vi "Wait.vi"(8 "error in (no error)":errorcluster, 10 "Wait":bool, 11 "Waiting Dialog View in":refnum<class "Waiting Dialog View.lvclass">) -> (0 "error out":errorcluster, 3 "Waiting Dialog View out":refnum<class "Waiting Dialog View.lvclass">)   [LabVIEW 2015, in "Waiting Dialog View.lvlib" / "Waiting Dialog View.lvclass"]
uses:
  Waiting Dialog View.lvclass
  UI Controller/UI Controller Messages/Hide Subpanel Msg/Hide Subpanel Msg.lvclass
  <vilib>/Utility/miscctls.llb/LVPositionTypeDef.ctl
  UI Controller/UI Controller Messages/Hide Subpanel Msg/Hide Subpanel Msg.lvclass/Hide Subpanel Msg.ctl
  <vilib>/ActorFramework/Actor/Actor.lvclass/Actor.ctl
  <vilib>/ActorFramework/Self-Addressed Msg/Self-Addressed Msg.lvclass/Self-Addressed Msg.ctl
  <vilib>/ActorFrameworkMVC/View Controller/View Controller Messages/Insert Subpanel Msg/Insert Subpanel Msg.lvclass/Insert Subpanel Msg.ctl
  <vilib>/ActorFramework/Message Enqueuer/Message Enqueuer.lvclass/Message Enqueuer.ctl
  <vilib>/ActorFrameworkMVC/View Controller/View Controller Messages/Move Subpanel Msg/Move Subpanel Msg.lvclass/Move Subpanel Msg.ctl
  <vilib>/ActorFramework/Message Enqueuer/Enqueue.vi
  <vilib>/ActorFramework/Message Priority Queue/Priority Enqueue.vi
  <vilib>/ActorFramework/Self-Addressed Msg/Self-Addressed Msg.lvclass
  <vilib>/ActorFrameworkMVC/View Controller/View Controller Messages/Insert Subpanel Msg/Insert Subpanel Msg.lvclass
  <vilib>/ActorFrameworkMVC/View Controller/View Controller Messages/Move Subpanel Msg/Move Subpanel Msg.lvclass
  <vilib>/ActorFramework/Actor/Actor.lvclass
panel:
  # "NOTICE -- YOU MUST LEAVE THIS NOTICE IN PLACE.\n\nCopyright (c) 2015, LIANG LIU Shawn.Liu.cn@gmail.com\nAll rights reserved.\n\nRedistribution and use in source and binary forms, with or without modification, are permitted provided that the following conditions are met:\n-Redistributions of source code must retain the above copyright notice, this list of conditions and the following disclaimer.\n-Redistributions in binary form must reproduce the above copyright notice, this list of conditions and the following disclaimer in the documentation and/or other materials provided with the distribution.\n-Neither the name of the eLp nor the names of its contributors may be used to endorse or promote products derived from this software without specific prior written permission.\n\nTHIS SOFTWARE IS PROVIDED BY THE COPYRIGHT HOLDERS AND CONTRIBUTORS \"AS IS\" AND ANY EXPRESS OR IMPLIED WARRANTIES, INCLUDING, BUT NOT LIMITED TO, THE IMPLIED WARRANTIES OF MERCHANTABILITY AND FITNESS FOR A PARTICULAR PURPOSE ARE DISCLAIMED. IN NO EVENT SHALL THE COPYRIGHT HOLDER OR CONTRIBUTORS BE LIABLE FOR ANY DIRECT, INDIRECT, INCIDENTAL, SPECIAL, EXEMPLARY, OR CONSEQUENTIAL DAMAGES (INCLUDING, BUT NOT LIMITED TO, PROCUREMENT OF SUBSTITUTE GOODS OR SERVICES; LOSS OF USE, DATA, OR PROFITS; OR BUSINESS INTERRUPTION) HOWEVER CAUSED AND ON ANY THEORY OF LIABILITY, WHETHER IN CONTRACT, STRICT LIABILITY, OR TORT (INCLUDING NEGLIGENCE OR OTHERWISE) ARISING IN ANY WAY OUT OF THE USE OF THIS SOFTWARE, EVEN IF ADVISED OF THE POSSIBILITY OF SUCH DAMAGE."
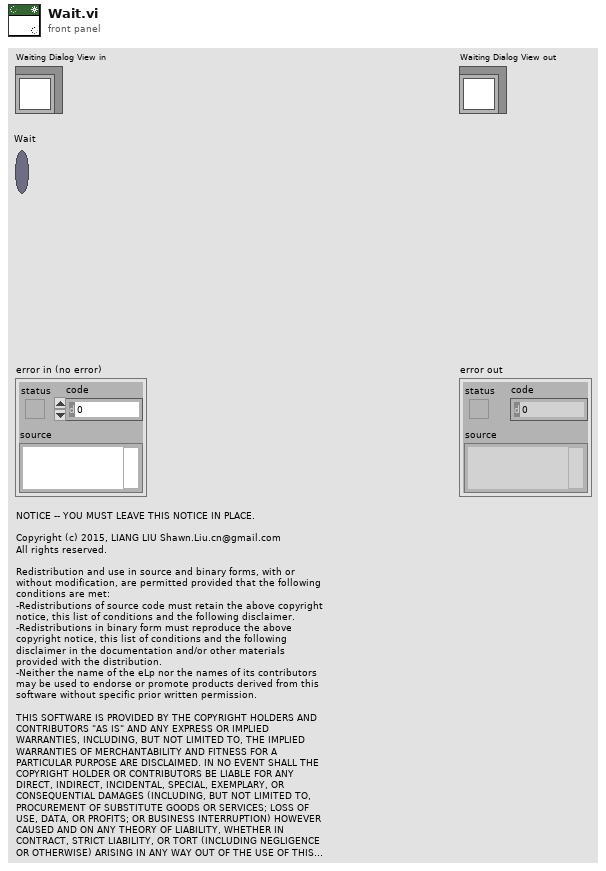
[diagram p1: front panel]
types:
  T1 = typedef "LVPositionTypeDef.ctl" = cluster{"Left":i32, "Top":i32}
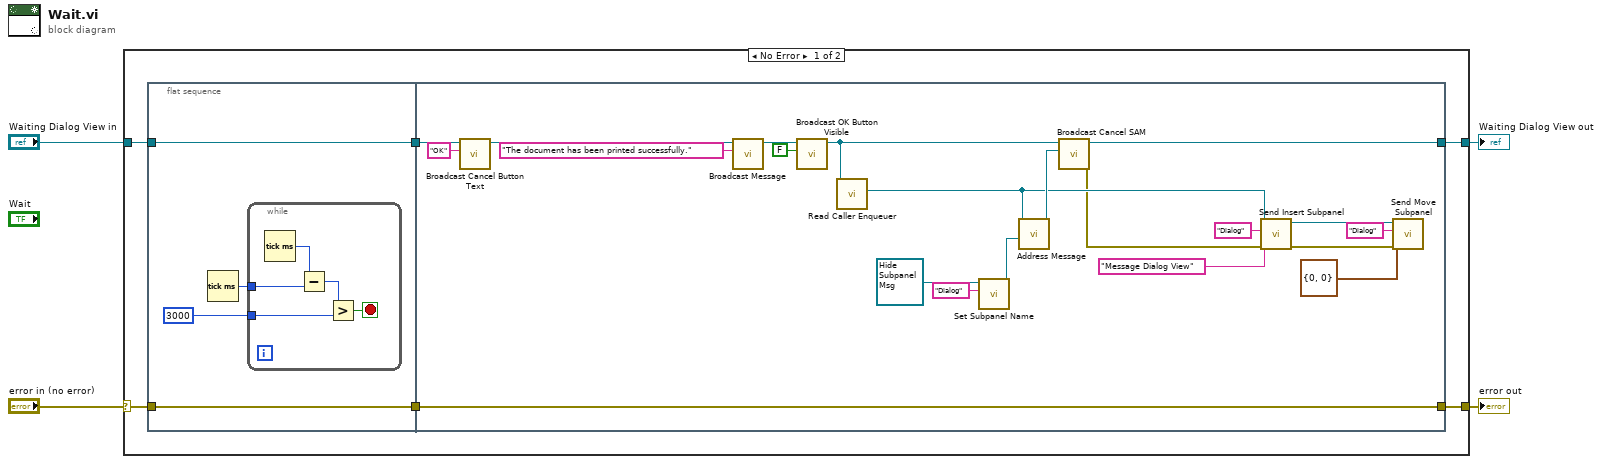
[diagram p0: block diagram]
diagram:
  n1 = case shown="No Error" "error in (no error)" {
    selector: "error in (no error)" -> [w6 w42]
    tunnel: "Waiting Dialog View in" -> [w8 w41]
    tunnel: [w7 w41] -> w3
    tunnel: [w5 w42] -> w1
    frame No Error {
      n2 = flat-sequence {
        tunnel: [w12] -> w10
        tunnel: w8 -> [w12]
        tunnel: [w11] -> w9
        tunnel: w6 -> [w11]
        tunnel: w10 -> [w40]
        tunnel: [w22] -> w7
        tunnel: w9 -> [w39]
        tunnel: [w39] -> w5
        frame #0 {
          n3 = Tick Count (ms)() -> (millisecond timer value=w14:u32)
          n4 = while {
            tunnel: w14 -> [w19]
            tunnel: u32 3000 ("y") -> [w17]
            stop <- w16 stop-if-true
            n5 = Tick Count (ms)() -> (millisecond timer value=w15:u32)
            n6 = Subtract(x=w15, y=w19) -> (x-y=w18:u32)
            n7 = Greater?(x=w18, y=w17) -> (0:w16:bool)
          }
        }
        frame #1 {
          n8 = call "Broadcast Cancel Button Text.vi"("Cancel Button Text"="OK", "Waiting Dialog View in"=w40) -> ("Waiting Dialog View out"=w38:refnum<class "Waiting Dialog View.lvclass">)  [unwired: 8 in, 1 out]
          n9 = call "Broadcast Message.vi"("Message"="The document has been printed successfully.", "Waiting Dialog View in"=w38) -> ("Waiting Dialog View out"=w36:refnum<class "Waiting Dialog View.lvclass">)  [unwired: 8 in, 1 out]
          n10 = call "Broadcast OK Button Visible.vi"("OK Button Visible"=FALSE, "Waiting Dialog View in"=w36) -> ("Waiting Dialog View out"=w23:refnum<class "Waiting Dialog View.lvclass">)  [unwired: 8 in, 1 out]
          n11 = call <vilib>:"Read Caller Enqueuer.vi"("Actor"=w23) -> ("Caller Enqueuer"=w25:refnum<class "Message Enqueuer.lvclass">)  [unwired: 10 in]
          n12 = call "Set Subpanel Name.vi"("Subpanel Name"="Dialog", "Hide Subpanel Msg in"=refnum<class "Hide Subpanel Msg.lvclass"> refnum ("View Controller.lvlib:Move Subpanel Msg.lvclass")) -> ("Hide Subpanel Msg out"=w21:refnum<class "Hide Subpanel Msg.lvclass">)  [unwired: 9 in]
          n13 = call <vilib>:"Address Message.vi"("Message"=w21, "Destination"=w25) -> ("Self-Addressed Message"=w32:refnum<class "Self-Addressed Msg.lvclass">)  [unwired: 9 in]
          n14 = call "Broadcast Cancel SAM.vi"("Cancel SAM"=w32, "Waiting Dialog View in"=w23) -> ("error out"=w24:errorcluster, "Waiting Dialog View out"=w22:refnum<class "Waiting Dialog View.lvclass">)  [unwired: 8 in]
          n15 = call <vilib>:"Send Insert Subpanel.vi"("error in (no error)"=w24, "View Name"="Message Dialog View" ("Subpanel Name"), "Subpanel Name"="Dialog", "Message Enqueuer"=w25) -> ("error out"=w29:errorcluster, "Message Enqueuer out"=w28:refnum<class "Message Enqueuer.lvclass">)  [unwired: 6 in]
          n16 = call <vilib>:"Send Move Subpanel.vi"("error in (no error)"=w29, "Position"=T1 {"Left"=0, "Top"=0}, "Subpanel Name"="Dialog", "Message Enqueuer"=w28) -> ()  [unwired: 6 in, 2 out]
        }
      }
    }
    frame Error {
    }
  }
  "error out" <- w1
  "Waiting Dialog View out" <- w3
